vi "rytimer_example.vi"() -> ()   [LabVIEW 2017]
uses:
  enqueue.ctl
  rytimer.lvclass
  rytimer.lvclass/rytimer.ctl
  <vilib>/Utility/error.llb/Error Cluster From Error Code.vi
  <vilib>/ErrorRing/Error Ring.xnode
panel:
  out "t2 time":timestamp
  out "t2 ms jitter chrt":dbl(graph)
  out "t2 ms dt":dbl
  out "t2 ms jitter":dbl
  out "t2 ms jitter avg":dbl
  out "t2 cnt":i32
  out "t1 ms jitter avg":dbl
  out "t1 ms jitter":dbl
  out "t1 time":timestamp
  out "t1 ms jitter chrt":dbl(graph)
  out "t1 cnt":i32
  out "t1 ms dt":dbl
  in  "t2 interval (ms)":u32=3000
  in  "t2 enqueue":T1=enum."front"
  in  "t2 auto-reset?":bool=TRUE
  in  "t1 auto-reset?":bool=TRUE
  in  "t1 enqueue":T1
  in  "t1 interval (ms)":u32=100
  in  "quit":bool
  # "Timer 1"
  # "Timer 2"
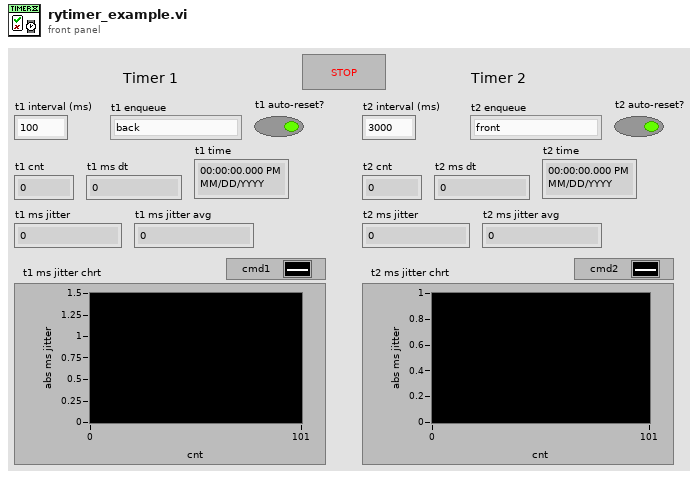
[diagram p1: front panel]
types:
  T1 = typedef "rytimer.lvclass/enqueue.ctl" = enum8{"back", "front", "back_if_absent", "front_if_absent"}
  T2 = cluster{"timer1":refnum<class "rytimer.lvclass">, "timer2":refnum<class "rytimer.lvclass">}
  T3 = enum8{"quit", "init1", "init2", "cmd1", "cmd2", "interval1", "interval2"}
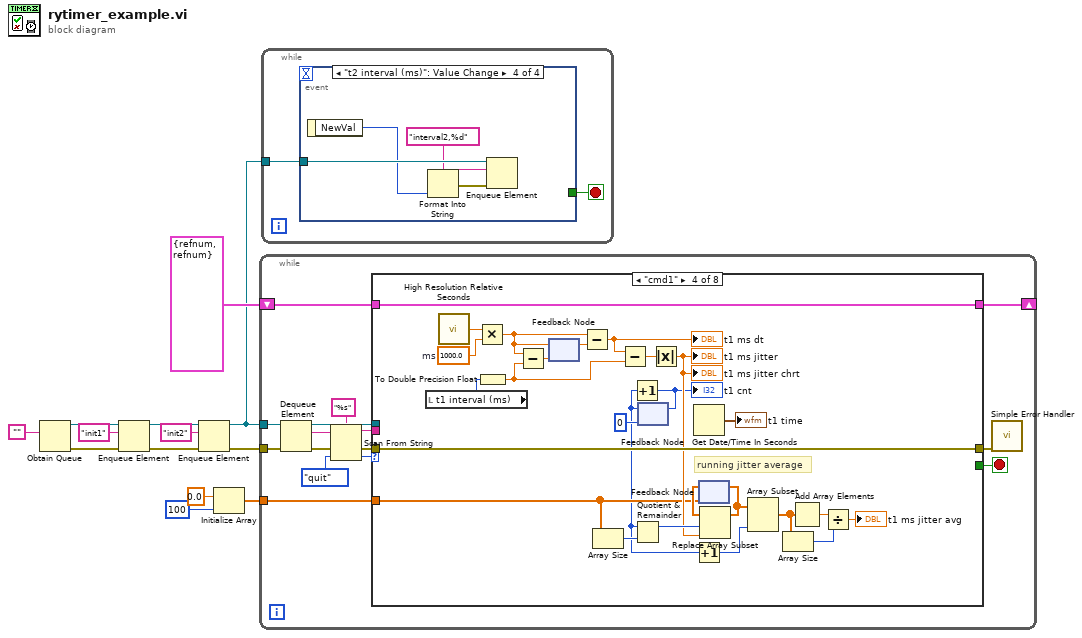
[diagram p0: block diagram]
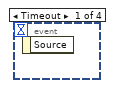
[diagram p2: hidden frame]
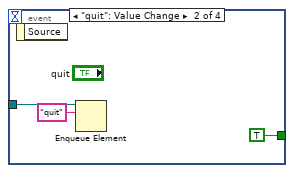
[diagram p3: hidden frame]
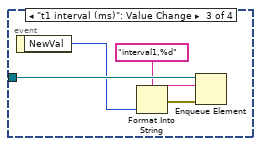
[diagram p4: hidden frame]
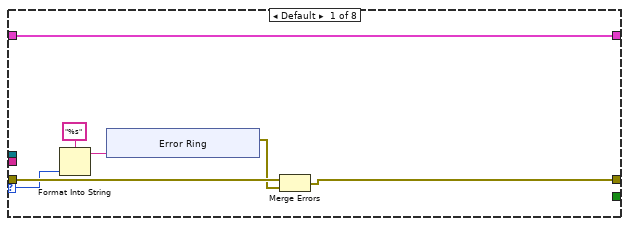
[diagram p5: hidden frame]
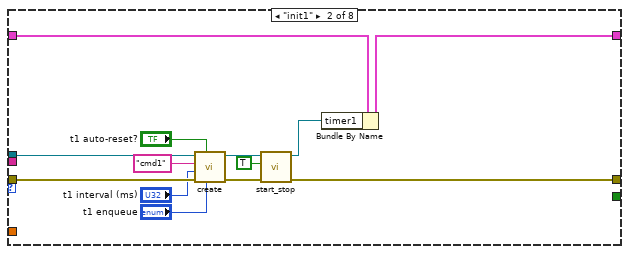
[diagram p6: hidden frame]
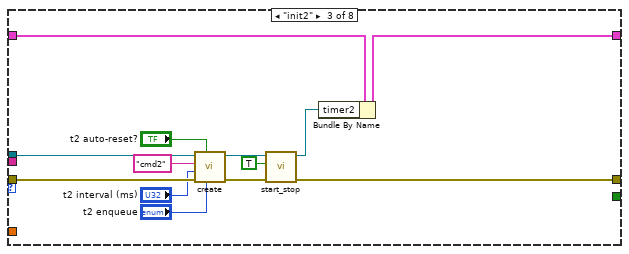
[diagram p7: hidden frame]
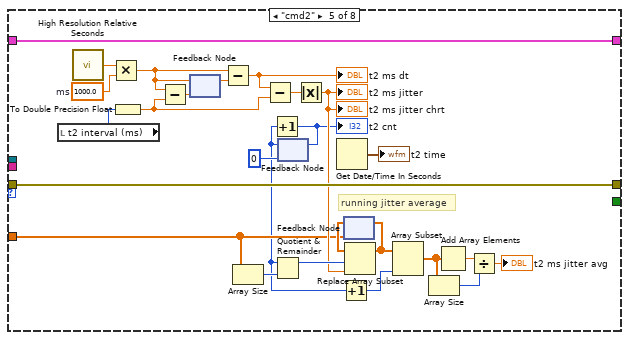
[diagram p8: hidden frame]
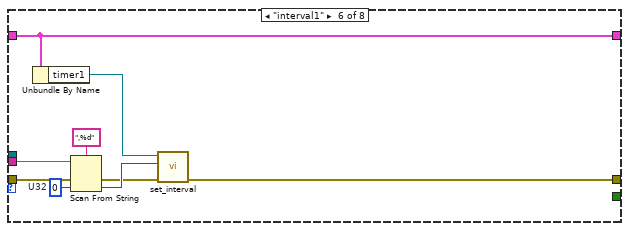
[diagram p9: hidden frame]
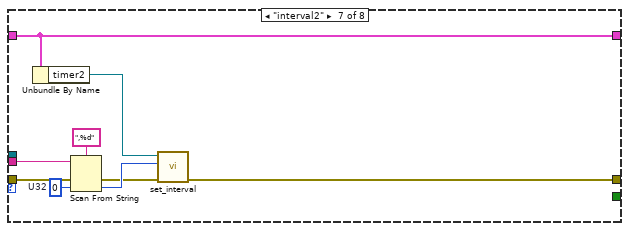
[diagram p10: hidden frame]
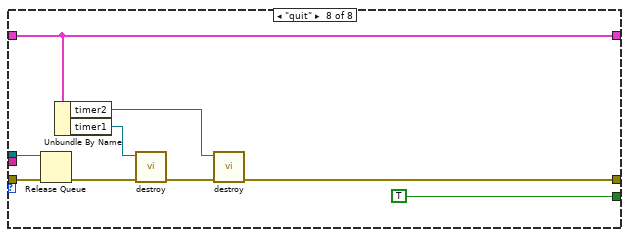
[diagram p11: hidden frame]
diagram:
  n1 = Obtain Queue(element data type="" ("Empty String Constant")) -> (queue out=w10:refnum<queue>, error out=w12:errorcluster)  [unwired: 4 in, 1 out]
  n2 = Enqueue Element(queue=w10, element="init1", error in (no error)=w12) -> (queue out=w6:refnum<queue>, error out=w11:errorcluster)  [unwired: 1 in, 1 out]
  n3 = Enqueue Element(queue=w6, element="init2", error in (no error)=w11) -> (queue out=w5:refnum<queue>, error out=w7:errorcluster)  [unwired: 1 in, 1 out]
  n4 = Initialize Array(0.0 ("element"), 100 ("dimension size")) -> (w1:dbl[])
  n5 = while {
    tunnel: w7 -> [w27]
    tunnel: w5 -> [w28]
    shift-right: [w24] -> _
    shift-left: T2 {"timer1"=refnum, "timer2"=refnum} ("data") -> [w23]
    tunnel: w1 -> [w14]
    stop <- w22 stop-if-true
    n6 = Dequeue Element(queue=w28, error in (no error)=w27) -> (queue out=w26:refnum<queue>, element=w19:string, error out=w25:errorcluster)  [unwired: 1 in, 1 out]
    n7 = Scan From String(format string="%s", input string=w19, error in=w25, default 1=T3."quit") -> (remaining string=w15:string, error out=w20:errorcluster, output 1=w16:T3)  [unwired: 1 in, 1 out]
    n8 = case shown="\"cmd1\"" w16 {
      selector: w16 -> [w30 _ _ _ _ _ _ _]
      tunnel: w26 -> [_ w54 w67 _ _ _ _ w146]
      tunnel: w20 -> [w35 w55 w68 w94 w120 w129 w138 w147]
      tunnel: [w33 w47 w60 w94 w120 w121 w130 w139] -> w21
      tunnel: [w34 w50 w63 w84 w110 w128 w137 w144] -> w24
      tunnel: w23 -> [w34 w53 w66 w84 w110 w128 w137 w144]
      tunnel: [_ _ _ _ _ _ _ TRUE] -> w22
      tunnel: w15 -> [_ _ _ _ _ w126 w135 _]
      tunnel: w14 -> [_ _ _ w82 w108 _ _ _]
      frame Default {
        n9 = Format Into String(format string="%s", w30) -> (resulting string=w31:string)  [unwired: 2 in, 1 out]
        n10 = xnode "Error Ring"("parameter 0"=w31) -> ("error out"=w32:errorcluster)
        n11 = Merge Errors(w35, w32) -> (w33:errorcluster)
      }
      frame "init1" {
        n12 = call "create.vi"("enqueue (back)"="t1 enqueue", "auto-reset? (T)"="t1 auto-reset?", "error in (no error)"=w55, "interval (1000 ms)"="t1 interval (ms)", "message (\"\"=Ignore)"="cmd1" ("message (\"\"=Ignore)"), "destination queue"=w54) -> ("error out"=w48:errorcluster, "timer"=w46:refnum<class "rytimer.lvclass">)  [unwired: 4 in]
        n13 = call "start_stop.vi"("error in (no error)"=w48, "start? (T)"=TRUE, "timer in"=w46) -> ("error out"=w47:errorcluster, "timer out"=w45:refnum<class "rytimer.lvclass">)  [unwired: 7 in]
        n14 = Bundle By Name(cluster=w53, "timer1"=w45) -> (w50:T2)
      }
      frame "init2" {
        n15 = call "create.vi"("enqueue (back)"="t2 enqueue", "auto-reset? (T)"="t2 auto-reset?", "error in (no error)"=w68, "interval (1000 ms)"="t2 interval (ms)", "message (\"\"=Ignore)"="cmd2" ("message (\"\"=Ignore)"), "destination queue"=w67) -> ("error out"=w61:errorcluster, "timer"=w59:refnum<class "rytimer.lvclass">)  [unwired: 4 in]
        n16 = call "start_stop.vi"("error in (no error)"=w61, "start? (T)"=TRUE, "timer in"=w59) -> ("error out"=w60:errorcluster, "timer out"=w58:refnum<class "rytimer.lvclass">)  [unwired: 7 in]
        n17 = Bundle By Name(cluster=w66, "timer2"=w58) -> (w63:T2)
      }
      frame "cmd1" {
        w89 = 1000.0  # ms
        # "running jitter average"
        n18 = local read "t1 interval (ms)"() -> (w80:u32)
        n19 = call <vilib>:"High Resolution Relative Seconds.vi"() -> ("relative seconds"=w77:dbl)
        n20 = Multiply(x=w77, y=w89) -> (x*y=w76:dbl)
        n21 = To Double Precision Float(number=w80) -> (double precision float=w79:dbl)
        n22 = Subtract(x=w76, y=w79) -> (x-y=w78:dbl)
        n23 = feedback #1(w78) -> (w90:dbl)
        n24 = feedback-in #1(w76) -> ()
        n25 = Subtract(x=w76, y=w90) -> (x-y=w75:dbl)
        "t1 ms dt" <- w75
        n26 = Array Size(array=w82) -> (size(s)=w81:i32)
        n27 = Subtract(x=w75, y=w79) -> (x-y=w86:dbl)
        n28 = feedback #2(0) -> (w70:i32)
        n29 = Increment(x=w70) -> (x+1=w69:i32)
        "t1 cnt" <- w69
        n30 = Quotient & Remainder(x=w70, y=w81) -> (x-y*floor(x/y)=w91:i32)  [unwired: 1 out]
        n31 = feedback-in #2(w69) -> ()
        n32 = Absolute Value(x=w86) -> (abs(x)=w85:dbl)
        "t1 ms jitter chrt" <- w85
        "t1 ms jitter" <- w85
        n33 = Get Date/Time In Seconds() -> (seconds since 1Jan1904=→"t1 time":timestamp)
        n34 = Increment(x=w70) -> (x+1=w71:i32)
        n35 = feedback #3(w82) -> (w83:dbl[])
        n36 = Replace Array Subset(array=w83, new element=w85, index=w91) -> (w74:dbl[])
        n37 = feedback-in #3(w74) -> ()
        n38 = Array Subset(array=w74, length=w71) -> (w73:dbl[])  [unwired: 1 in]
        n39 = Array Size(array=w73) -> (size(s)=w72:i32)
        n40 = Add Array Elements(numeric array=w73) -> (sum=w88:dbl)
        n41 = Divide(x=w88, y=w72) -> (x/y=→"t1 ms jitter avg":dbl)
      }
      frame "cmd2" {
        w103 = 1000.0  # ms
        # "running jitter average"
        n42 = local read "t2 interval (ms)"() -> (w111:u32)
        n43 = call <vilib>:"High Resolution Relative Seconds.vi"() -> ("relative seconds"=w102:dbl)
        n44 = Multiply(x=w102, y=w103) -> (x*y=w101:dbl)
        n45 = To Double Precision Float(number=w111) -> (double precision float=w106:dbl)
        n46 = Subtract(x=w101, y=w106) -> (x-y=w105:dbl)
        n47 = feedback #4(w105) -> (w116:dbl)
        n48 = feedback-in #4(w101) -> ()
        n49 = Subtract(x=w101, y=w116) -> (x-y=w104:dbl)
        "t2 ms dt" <- w104
        n50 = Array Size(array=w108) -> (size(s)=w107:i32)
        n51 = Subtract(x=w104, y=w106) -> (x-y=w113:dbl)
        n52 = feedback #5(0) -> (w96:i32)
        n53 = Increment(x=w96) -> (x+1=w99:i32)
        "t2 cnt" <- w99
        n54 = Quotient & Remainder(x=w96, y=w107) -> (x-y*floor(x/y)=w117:i32)  [unwired: 1 out]
        n55 = feedback-in #5(w99) -> ()
        n56 = Absolute Value(x=w113) -> (abs(x)=w112:dbl)
        "t2 ms jitter chrt" <- w112
        "t2 ms jitter" <- w112
        n57 = Get Date/Time In Seconds() -> (seconds since 1Jan1904=→"t2 time":timestamp)
        n58 = Increment(x=w96) -> (x+1=w95:i32)
        n59 = feedback #6(w108) -> (w109:dbl[])
        n60 = Replace Array Subset(array=w109, new element=w112, index=w117) -> (w100:dbl[])
        n61 = feedback-in #6(w100) -> ()
        n62 = Array Subset(array=w100, length=w95) -> (w98:dbl[])  [unwired: 1 in]
        n63 = Array Size(array=w98) -> (size(s)=w97:i32)
        n64 = Add Array Elements(numeric array=w98) -> (sum=w115:dbl)
        n65 = Divide(x=w115, y=w97) -> (x/y=→"t2 ms jitter avg":dbl)
      }
      frame "interval1" {
        w124 = u32 0  # U32
        n66 = Unbundle By Name(w128) -> ("timer1"=w127:refnum<class "rytimer.lvclass">)
        n67 = Scan From String(format string=",%d", input string=w126, error in=w129, default 1=w124) -> (error out=w122:errorcluster, output 1=w123:u32)  [unwired: 1 in, 2 out]
        n68 = call "set_interval.vi"("error in (no error)"=w122, "interval (1000 ms)"=w123, "timer in"=w127) -> ("error out"=w121:errorcluster)  [unwired: 7 in, 1 out]
      }
      frame "interval2" {
        w133 = u32 0  # U32
        n69 = Unbundle By Name(w137) -> ("timer2"=w136:refnum<class "rytimer.lvclass">)
        n70 = Scan From String(format string=",%d", input string=w135, error in=w138, default 1=w133) -> (error out=w131:errorcluster, output 1=w132:u32)  [unwired: 1 in, 2 out]
        n71 = call "set_interval.vi"("error in (no error)"=w131, "interval (1000 ms)"=w132, "timer in"=w136) -> ("error out"=w130:errorcluster)  [unwired: 7 in, 1 out]
      }
      frame "quit" {
        n72 = Release Queue(queue=w146, error in (no error)=w147) -> (error out=w143:errorcluster)  [unwired: 1 in, 2 out]
        n73 = Unbundle By Name(w144) -> ("timer2"=w140:refnum<class "rytimer.lvclass">, "timer1"=w142:refnum<class "rytimer.lvclass">)
        n74 = call "destroy.vi"("error in (no error)"=w143, "timer"=w142) -> ("error out"=w141:errorcluster)  [unwired: 9 in]
        n75 = call "destroy.vi"("error in (no error)"=w141, "timer"=w140) -> ("error out"=w139:errorcluster)  [unwired: 9 in]
      }
    }
    n76 = call <vilib>:"Simple Error Handler.vi"("error in (no error)"=w21) -> ()  [unwired: 4 in, 5 out]
  }
  n77 = while {
    tunnel: w5 -> [w149]
    stop <- w148 stop-if-true
    n78 = event shown="[3] \"t2 interval (ms)\": Value Change" {
      selector: _ -> [_ _ _ _]
      dyn-events: _ -> [_ _ _ _]
      timeout: _ -> [_ _ _ _]
      tunnel: w149 -> [_ w151 w157 w162]
      tunnel: [_ TRUE _ _] -> w148
      event Timeout {
        n79 = event-data() -> ()  [unwired: 1 in, 1 out]
      }
      event "quit": Value Change {
        n80 = event-data() -> ()  [unwired: 1 in, 1 out]
        n81 = Enqueue Element(queue=w151, element="quit") -> ()  [unwired: 2 in, 3 out]
      }
      event "t1 interval (ms)": Value Change {
        n82 = event-data() -> ("NewVal"=w153:u32)  [unwired: 1 in]
        n83 = Format Into String(format string="interval1,%d" ("element"), w153) -> (resulting string=w155:string, error out=w156:errorcluster)  [unwired: 2 in]
        n84 = Enqueue Element(queue=w157, element=w155, error in (no error)=w156) -> ()  [unwired: 1 in, 3 out]
      }
      event "t2 interval (ms)": Value Change {
        n85 = event-data() -> ("NewVal"=w158:u32)  [unwired: 1 in]
        n86 = Format Into String(format string="interval2,%d" ("element"), w158) -> (resulting string=w160:string, error out=w161:errorcluster)  [unwired: 2 in]
        n87 = Enqueue Element(queue=w162, element=w160, error in (no error)=w161) -> ()  [unwired: 1 in, 3 out]
      }
    }
  }
